vi "Camera_Histogram.vi"(2 "SRV In":string) -> (4 "SRV Out":string="169.254.0.10")   [LabVIEW 2009]
panel:
  out "data out":string
  # "This LabVIEW item is deprecated.\n\nIt is believed to be unused and will be removed in a future version of SRV."
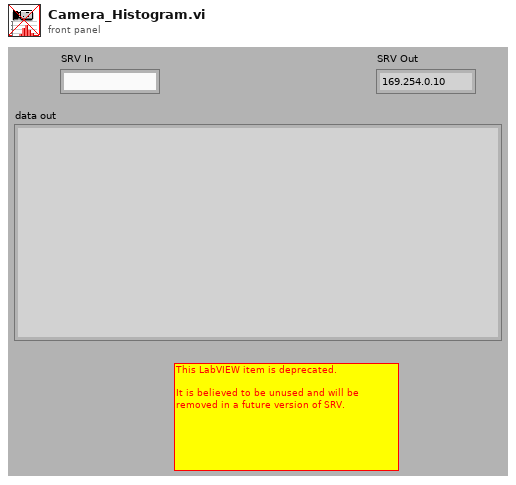
[diagram p1: front panel]
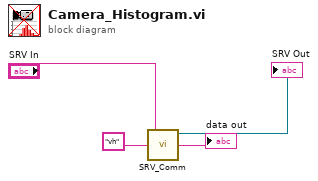
[diagram p0: block diagram]
diagram:
  n1 = call "SRV_Comm.vi"("Command Sent"="vh", "SRV In"="SRV In") -> ("Reply"=→"data out":string, "SRV Out"=→"SRV Out":refnum<k5>)  [unwired: 1 in, 1 out]
